vi "Set LowLimit.vi"(8 "error in":errorcluster, 10 "Value.lvclass":refnum<class "Value.lvclass">, 11 "Object Type in":refnum<class "ARRAY.lvclass">) -> (0 "error out":errorcluster, 3 "Object Type out":refnum<class "ARRAY.lvclass">)   [LabVIEW 2024, in "Electronic Datasheet.lvlib" / "ARRAY.lvclass"]
uses:
  ARRAY.lvclass
  ARRAY.lvclass/ARRAY.ctl
  Value/Value.lvclass
  Electronic Datasheet.lvlib
  D:/git/EDS-File-Viewer/Core/Object Type/Object Type Base.lvclass
  D:/git/EDS-File-Viewer/Core/ARRAY/ARRAY.lvclass
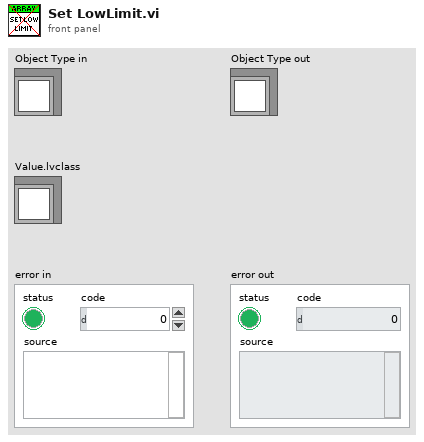
[diagram p1: front panel]
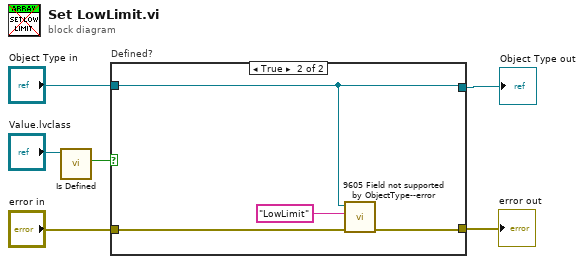
[diagram p0: block diagram]
diagram:
  n1 = call "Is Defined.vi"("Value in"="Value.lvclass") -> ("Is Defined?"=w1:bool)  [unwired: 9 in, 1 out]
  n2 = case "Defined?" shown="True" w1 {
    tunnel: [w8 w11] -> w5
    tunnel: "Object Type in" -> [w7 w9]
    tunnel: [w7 w9] -> w4
    tunnel: "error in" -> [w8 w12]
    frame False {
    }
    frame True {
      n3 = call "9605 Field not supported by ObjectType--error.vi"("error in"=w12, "Field Name"="LowLimit" ("Field name"), "Object Type Base"=w9) -> ("error out"=w11:errorcluster)  [unwired: 8 in]
    }
  }
  "Object Type out" <- w4
  "error out" <- w5
